vi "对中.vi"(8 "error in (no error)":errorcluster caption="错误输入（无错误）", 11 "信号数据":dbl[][](array[numeric])) -> (0 "error out":errorcluster caption="错误输出")   [LabVIEW 2015, in "Logging.lvlib"]
uses:
  Logging.lvlib
panel:
  out "偏差角度":dbl format="%0.2f"
  out "偏差扭矩":dbl format="%0.2f"
  in  "取消按钮":bool
  in  "确定按钮":bool
  # "对称测量结果"
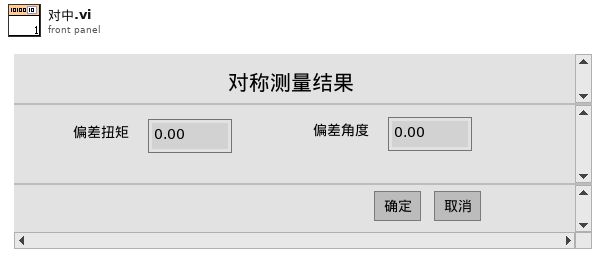
[diagram p1: front panel]
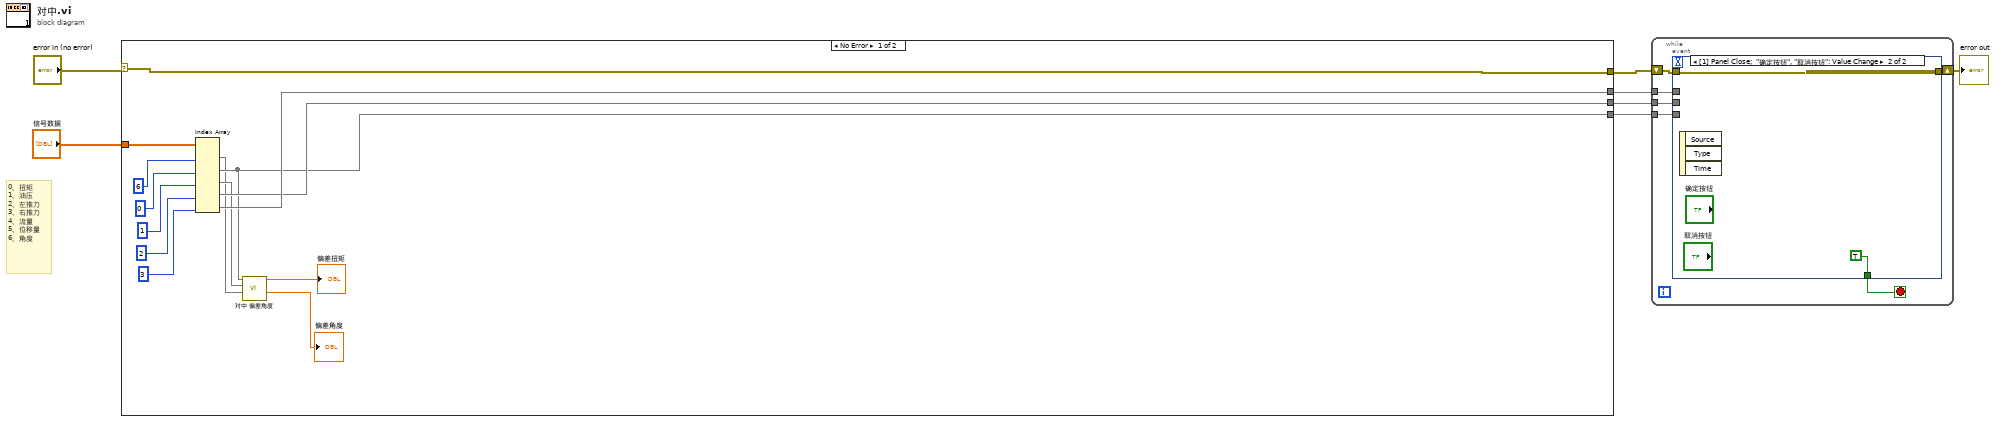
[diagram p0: block diagram]
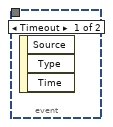
[diagram p2: hidden frame]
diagram:
  # "0、扭矩\n1、油压\n2、左推力\n3、右推力\n4、流量\n5、位移量\n6、角度"
  n1 = case shown="No Error" "error in (no error)" {
    selector: "error in (no error)" -> [w20 w22]
    tunnel: "信号数据" -> [w21 _]
    tunnel: [w20 w22] -> w5
    tunnel: [w19 _] -> w3
    tunnel: [w18 _] -> w2
    tunnel: [w17 _] -> w1
    frame No Error {
      n2 = Index Array(array=w21, index (col) #1=6 ("禁用的索引 (列)"), index (col) #2=0 ("索引 (行)"), index (col) #3=1 ("索引 (行)"), index (col) #4=2 ("索引 (行)"), index (col) #5=3 ("索引 (行)")) -> (element #1=w15:dbl[], element #2=w17:dbl[], element #3=w16:dbl[], element #4=w18:dbl[], element #5=w19:dbl[])  [unwired: 5 in]
      n3 = call "对中 偏差角度.vi"("角度"=w15, "油压"=w16, "扭矩"=w17) -> ("偏差角度"=→"偏差角度":dbl, "偏差扭矩"=→"偏差扭矩":dbl)  [unwired: 7 in]
    }
    frame Error {
    }
  }
  n4 = while {
    shift-right: [w27] -> w4
    shift-left: w5 -> [w28]
    tunnel: w3 -> [w24]
    tunnel: w2 -> [w23]
    tunnel: w1 -> [w25]
    stop <- w26 stop-if-true
    n5 = event shown="[1] Panel Close;  \"确定按钮\", \"取消按钮\": Value Change" {
      selector: _ -> [_ _]
      dyn-events: _ -> [_ _]
      timeout: _ -> [_ _]
      tunnel: w28 -> [_ w30]
      tunnel: [_ w30] -> w27
      tunnel: [_ TRUE] -> w26
      tunnel: w25 -> [_ _]
      tunnel: w24 -> [_ _]
      tunnel: w23 -> [_ _]
      event Timeout {
        n6 = event-data() -> ()  [unwired: 1 in, 3 out]
      }
      event Panel Close; "确定按钮", "取消按钮": Value Change {
        n7 = event-data() -> ()  [unwired: 1 in, 3 out]
      }
    }
  }
  "error out" <- w4
